vi "Test Read Ref.vi"() -> ()   [LabVIEW 2020]
uses:
  src/ClientApp1/ClientApp1/ClientApp1.lvclass
  C:/Users/dzoni/Documents/GitHub/client/src/ClientBase/ClientBase.lvclass
  src/ClientBase/ClientBase.lvclass
  src/ClientApp1/ClientApp1Lib.lvlib
panel:
  out "ID":string
  out "Port":u16
  out "Data 2":string
  out "Data":string
  out "Address":string
  out "error out":errorcluster
  # "56 - The network operation exceeded the user-specified or system time limit."
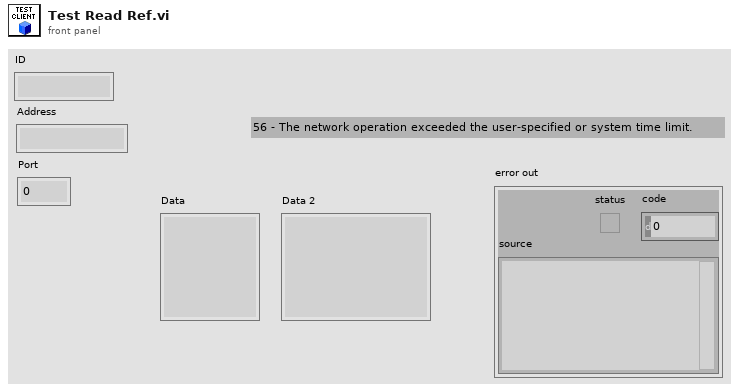
[diagram p1: front panel]
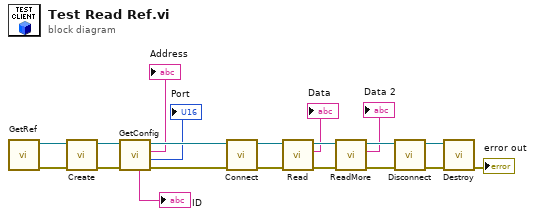
[diagram p0: block diagram]
diagram:
  n1 = call "GetRef.vi"() -> ("error out"=w1:errorcluster, "ClientApp1 out"=w2:refnum<class "ClientApp1.lvclass">)  [unwired: 10 in]
  n2 = call-dynamic "Create.vi"("error in (no error)"=w1, "ClientApp1 in"=w2) -> ("error out"=w11:errorcluster, "ClientApp1 out"=w14:refnum<class "ClientApp1.lvclass">)  [unwired: 8 in]
  n3 = call "GetConfig.vi"("error in (no error)"=w11, "ClientBase in"=w14) -> ("error out"=w10:errorcluster, "Port"=→"Port":u16, "Address"=→"Address":string, "ClientBase out"=w13:refnum<class "ClientApp1.lvclass">, "ID"=→"ID":string)  [unwired: 5 in]
  n4 = call-dynamic "Connect.vi"("error in (no error)"=w10, "ClientBase in"=w13) -> ("error out"=w9:errorcluster, "ClientBase out"=w12:refnum<class "ClientApp1.lvclass">)  [unwired: 8 in]
  n5 = call-dynamic "Read.vi"("error in (no error)"=w9, "ClientBase in"=w12) -> ("error out"=w8:errorcluster, "Data"=→"Data":string, "ClientBase out"=w15:refnum<class "ClientApp1.lvclass">)  [unwired: 7 in]
  n6 = call "ReadMore.vi"("error in (no error)"=w8, "ClientApp1 in"=w15) -> ("error out"=w19:errorcluster, "Data"=→"Data 2":string, "ClientApp1 out"=w20:refnum<class "ClientApp1.lvclass">)  [unwired: 7 in]
  n7 = call-dynamic "Disconnect.vi"("error in (no error)"=w19, "ClientBase in"=w20) -> ("error out"=w18:errorcluster, "ClientBase out"=w17:refnum<class "ClientApp1.lvclass">)  [unwired: 8 in]
  n8 = call-dynamic "Destroy.vi"("error in (no error)"=w18, "ClientBase in"=w17) -> ("error out"=→"error out":errorcluster)  [unwired: 9 in]
